vi "Close.vi"(8 "error in (no error)":errorcluster caption="entrée d'erreur (pas d'erreur)", 11 "Cryptographic Hash_SHA256 en entrée":refnum<class "Cryptographic Hash_SHA256.lvclass">) -> (0 "error out":errorcluster caption="sortie d'erreur", 3 "Cryptographic Hash_SHA256 en sortie":refnum<class "Cryptographic Hash_SHA256.lvclass">)   [LabVIEW 2020, in "Library Cryptographic Hash.lvlib" / "Cryptographic Hash_SHA256.lvclass"]
uses:
  Cryptographic Hash_SHA256.lvclass
  Cryptographic Hash_SHA256.lvclass/Cryptographic Hash_SHA256.ctl
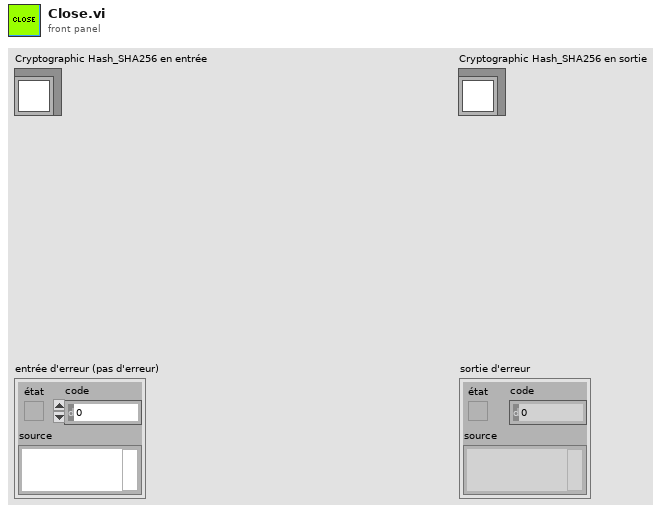
[diagram p1: front panel]
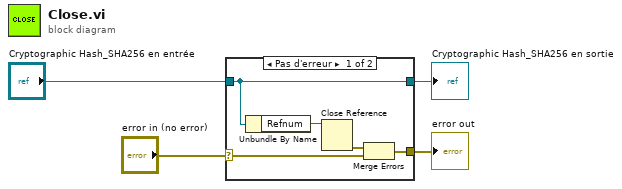
[diagram p0: block diagram]
diagram:
  n1 = case shown="Pas d'erreur" "error in (no error)" {
    selector: "error in (no error)" -> [w8 w11]
    tunnel: [w7 w11] -> w3
    tunnel: [w6 w10] -> w1
    tunnel: "Cryptographic Hash_SHA256 en entrée" -> [w6 w10]
    frame No Error {
      n2 = Unbundle By Name(w6) -> ("Refnum"=w5:refnum<k24>)
      n3 = Close Reference(reference=w5) -> (error out=w9:errorcluster)  [unwired: 1 in]
      n4 = Merge Errors(w9, w8) -> (w7:errorcluster)
    }
    frame Error {
    }
  }
  "error out" <- w3
  "Cryptographic Hash_SHA256 en sortie" <- w1
